vi "From Value.vi"(8 "error in (no error)":errorcluster, 10 "PV Data in":refnum<class "PV Data.lvclass">, 11 "NT Enum in":refnum<class "NT Enum.lvclass">) -> (0 "error out":errorcluster, 2 "PV Data out":refnum<class "PV Data.lvclass">, 3 "NT Enum out":refnum<class "NT Enum.lvclass">)   [LabVIEW 2020, in "PV Access.lvlib" / "PV Data.lvlib" / "NT Enum.lvclass"]
uses:
  NT Enum.lvclass
  PV Data/PV Data.lvclass
  NT Base/NT Base.lvclass
  NT Enum.lvclass/NT Enum.ctl
  PV Data/Read Field (String Array).vi
  PV Data/Read Field (I32).vi
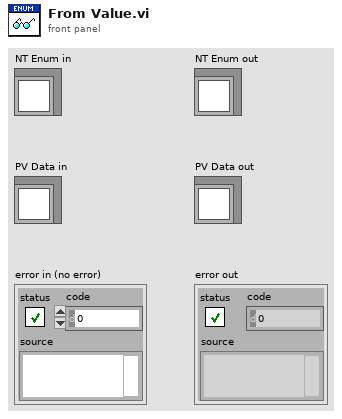
[diagram p1: front panel]
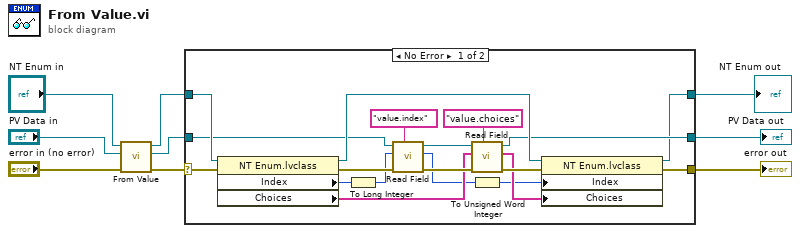
[diagram p0: block diagram]
diagram:
  n1 = call-parent "From Value.vi"("error in (no error)"="error in (no error)", "PV Data in"="PV Data in", "NT Base in"="NT Enum in") -> ("error out"=w1:errorcluster, "PV Data out"=w2:refnum<class "PV Data.lvclass">, "NT Base out"=w3:refnum<class "NT Enum.lvclass">)  [unwired: 6 in]
  n2 = case shown="No Error" w1 {
    selector: w1 -> [w24 w29]
    tunnel: [w16 w29] -> w9
    tunnel: [w18 w30] -> w8
    tunnel: [w17 w31] -> w7
    tunnel: w2 -> [w23 w30]
    tunnel: w3 -> [w28 w31]
    frame No Error {
      n3 = property class="NT Enum.lvclass"(reference=w28, error in=w24) -> (reference out=w25:refnum<class "NT Enum.lvclass">, error out=w26:errorcluster, "Index"=w13:u16, "Choices"=w15:string[])
      n4 = To Long Integer(number=w13) -> (32bit integer=w12:i32)
      n5 = call-poly "Read Field.vi"("field name"="value.index", "error in (no error)"=w26, "default"=w12, "PV Data in"=w23) -> ("error out"=w21:errorcluster, "value"=w11:i32, "PV Data out"=w19:refnum<class "PV Data.lvclass">)  [unwired: 5 in]
      n6 = call-poly "Read Field.vi"("field name"="value.choices", "error in (no error)"=w21, "default"=w15, "PV Data in"=w19) -> ("error out"=w20:errorcluster, "value"=w14:string[], "PV Data out"=w18:refnum<class "PV Data.lvclass">)  [unwired: 5 in]
      n7 = To Unsigned Word Integer(number=w11) -> (unsigned 16bit integer=w10:u16)
      n8 = property class="NT Enum.lvclass"(reference=w25, error in=w20, "Index"=w10, "Choices"=w14) -> (reference out=w17:refnum<class "NT Enum.lvclass">, error out=w16:errorcluster)
    }
    frame Error {
    }
  }
  "error out" <- w9
  "NT Enum out" <- w7
  "PV Data out" <- w8
